vi "BotSpeakSerial_Init.vi"(3 "Bot Settings in":T1) -> (0 "error out":errorcluster, 1 "Bot Settings out":T1)   [LabVIEW 2014]
uses:
  <userlib>/botspeakLib/VIs/Direct/BotSpeak_Control.ctl
  <vilib>/Instr/_visa.llb/VISA Configure Serial Port (Instr).vi
  <userlib>/botspeakLib/VIs/SubVIs/BotSpeak_Globals.vi
panel:
  out "Address":string
  out "StartupWait":i32
  out "Com Protocol":string
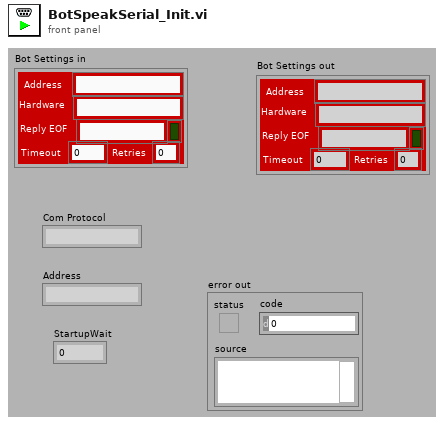
[diagram p1: front panel]
types:
  T1 = typedef "BotSpeak_Control.ctl" = cluster{"Address":string, "Reply EOF":string, "Hardware":string, "Retries":i8, "Timeout":i32, "Open?":bool}
  T2 = typedef "BotSpeak.HardwareSpecs.ctl" = cluster{"Hardware Name":string, "Hardware URL":string, "ComType":enum16{"Undefined", "HTTP", "Serial", "TCPIP", "Console"}, "TCP Port":i32, "DefaultAddress":string, "Retries":i32, "Translate":enum16{"None", "Tiny", "URAPI"}, "MaxScriptSize":i32, "MaxVarNumber":i32, "StartupWait":i32, "Patience":i32, "Startup Patience":i32, "Hardware Help":string, "Com Protocol":string, "Translator":cluster{"BotSpeak CMD":string, "CMD out":string}[], "Init Code":string, "Variable Format":enum16{"INT", "FLOAT", "FIXED"}, "username":string, "password":string}
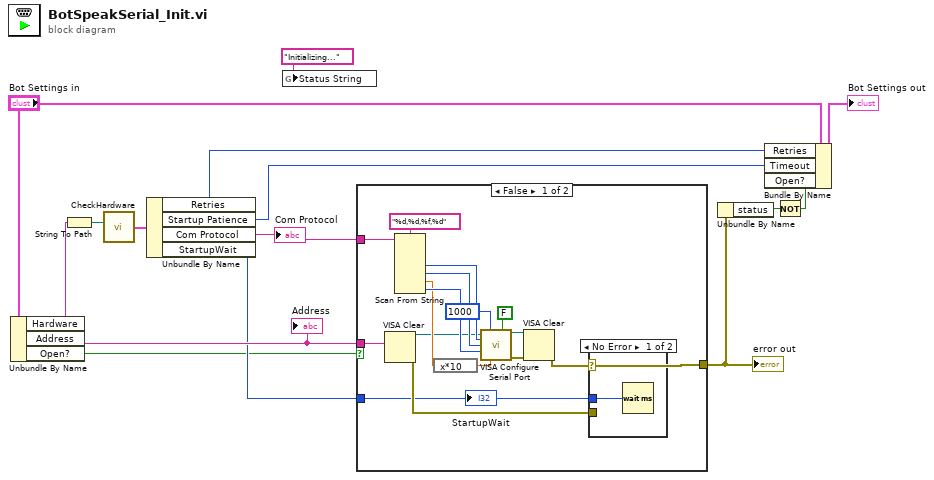
[diagram p0: block diagram]
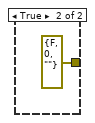
[diagram p3: hidden frame]
diagram:
  n1 = Unbundle By Name("Bot Settings in") -> ("Hardware"=w15:string, "Address"=w14:string, "Open?"=w4:bool)
  "Address" <- w14
  n2 = String To Path(string=w15) -> (path=w5:path)
  n3 = call <userlib>:"CheckHardware.vi"("Hardware"=w5) -> ("HardwareSpecs"=w13:T2)  [unwired: 2 in]
  n4 = Unbundle By Name(w13) -> ("Retries"=w7:i32, "Startup Patience"=w8:i32, "Com Protocol"=w12:string, "StartupWait"=w11:i32)
  "Com Protocol" <- w12
  n5 = global write "BotSpeak_Globals.vi" "Status String"("Initializing..." ("Status String")) -> ()
  n6 = case shown="False" w4 {
    tunnel: w14 -> [w20 _]
    tunnel: w12 -> [w19 _]
    tunnel: w11 -> [w18 _]
    tunnel: [w16 errorcluster {"status"=FALSE, "code"=0, "source"=""} ("error out")] -> w3
    frame False {
      n7 = VISA Clear(VISA resource name=w20) -> (VISA resource name out=w24:refnum<visa-resource-name>, error out=w22:errorcluster)  [unwired: 1 in]
      n8 = Scan From String(format string="%d,%d,%f,%d", input string=w19) -> (output 1=w27:i32, output 2=w28:i32, output 3=w29:dbl, output 4=w30:i32)  [unwired: 6 in, 3 out]
      n9 = expression code="x*10"(w29) -> (w31:dbl)
      n10 = call-poly "VISA Configure Serial Port"("VISA resource name"=w24, "timeout (10sec)"=u32 1000, "Enable Termination\nChar (T)"=FALSE ("Enable Termination\nChar (T)"), "baud rate (9600)"=w27, "data bits (8)"=w28, "parity (0:none)"=w30, "stop bits (10: 1 bit)"=w31) -> ("VISA resource name out"=w21:refnum<visa-resource-name>, "error out"=w17:errorcluster)  [unwired: 7 in]
      n11 = VISA Clear(VISA resource name=w21, error in (no error)=w17) -> (error out=w16:errorcluster)  [unwired: 1 out]
      n12 = case shown="No Error" w16 {
        tunnel: w18 -> [w32 _]
        tunnel: w22 -> [_ _]
        frame No Error {
          n13 = Wait (ms)(milliseconds to wait=w32) -> ()  [unwired: 1 out]
        }
        frame Error {
        }
      }
      "StartupWait" <- w18
    }
    frame True {
    }
  }
  "error out" <- w3
  n14 = Unbundle By Name(w3) -> ("status"=w1:bool)
  n15 = Not(x=w1) -> (.not. x?=w2:bool)
  n16 = Bundle By Name(cluster="Bot Settings in", "Retries"=w7, "Timeout"=w8, "Open?"=w2) -> (→"Bot Settings out":T1)
